vi "List.vi"(8 "error in (no error)":errorcluster, 11 "BCReg":refnum<data-value>) -> (0 "error out":errorcluster, 1 "First(all)":bool[](array[boolean]), 2 "Found?":bool, 3 "BCReg":refnum<data-value>, 4 "BC IDs":i32[](array[numeric]), 5 "Instance Names":string[](array[string]))   [LabVIEW 2017, in "BusController.lvlib" / "BCReg.lvclass"]
uses:
  BCReg.lvclass
  BCReg.lvclass/BCReg.ctl
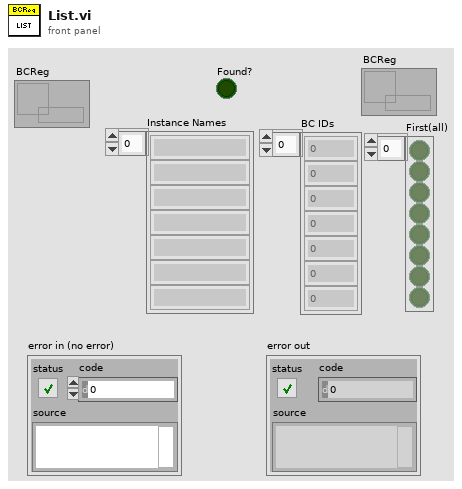
[diagram p1: front panel]
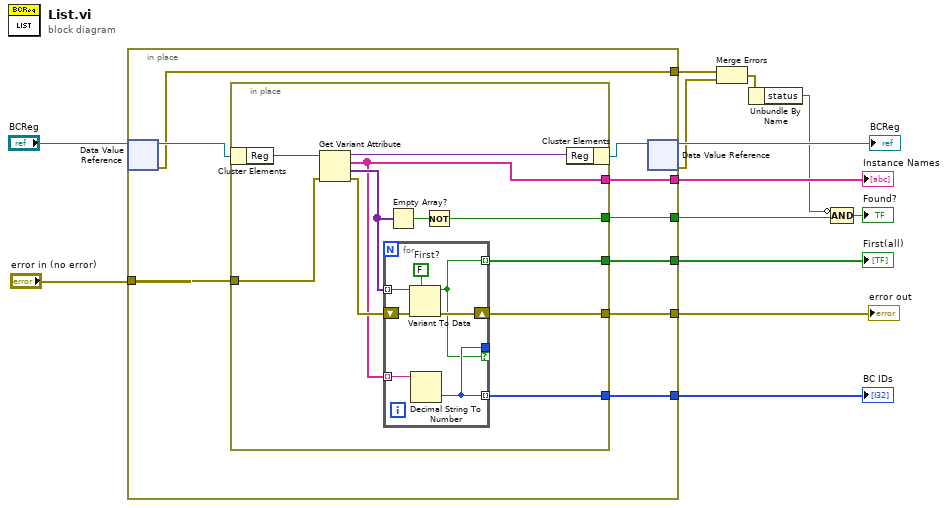
[diagram p0: block diagram]
diagram:
  n1 = in-place {
    in-place-border: [w22] -> w3
    in-place-border: [w21] -> w10
    in-place-border: "error in (no error)" -> [w20]
    in-place-border: [w19] -> w7
    in-place-border: [w18] -> w8
    in-place-border: [w17] -> w9
    in-place-border: [w14] -> w6
    n2 = in-place-dvr #1("BCReg") -> (w15:refnum<class "BCReg.lvclass">, w14:errorcluster)
    n3 = in-place {
      in-place-border: [w28] -> w22
      in-place-border: [w27] -> w21
      in-place-border: w20 -> [w26]
      in-place-border: [w25] -> w19
      in-place-border: [w24] -> w18
      in-place-border: [w23] -> w17
      n4 = in-place-cluster #2(w15) -> ("Reg"=w33:variant)
      n5 = Get Variant Attribute(Variant=w33, error in=w26) -> (duplicate Variant=w32:variant, names=w25:string[], values=w29:variant[], error out=w31:errorcluster)  [unwired: 2 in]
      n6 = for {
        tunnel: w25 -> [w40] mode=indexing
        tunnel: [w35] -> w24 mode=indexing
        tunnel: w29 -> [w39] mode=indexing
        shift-right: [w36] -> w27
        shift-left: w31 -> [w37]
        tunnel: [w34] -> w23 mode=indexing
        tunnel: [w35] -> _ if=w34
        w38 = FALSE  # First?
        n7 = Variant To Data(error in=w37, type=w38, Variant=w39) -> (data=w34:bool, error out=w36:errorcluster)
        n8 = Decimal String To Number(string=w40) -> (number=w35:i32)  [unwired: 2 in, 1 out]
      }
      n9 = Empty Array?(array=w29) -> (empty?=w30:bool)
      n10 = Not(x=w30) -> (.not. x?=w28:bool)
      n11 = in-place-cluster #2("Reg"=w32) -> (w16:refnum<class "BCReg.lvclass">)
    }
    n12 = in-place-dvr #1(w16) -> (→"BCReg":refnum<data-value>, w5:errorcluster)
  }
  "error out" <- w10
  "First(all)" <- w9
  "BC IDs" <- w8
  "Instance Names" <- w7
  n13 = Merge Errors(w6, w5) -> (w4:errorcluster)
  n14 = Unbundle By Name(w4) -> ("status"=w1:bool)
  n15 = Compound Arithmetic op=AND(invert w1, w3) -> (→"Found?":bool)
